vi "Auto Wheel Offsets.vi"() -> ()   [LabVIEW 2015]
uses:
  <vilib>/Rock Robotics/Network Tables/NT Write Number.vi
panel:
  out "FR Offset":dbl
  out "FL Offset":dbl
  out "BR Offset":dbl
  out "BL Offset":dbl
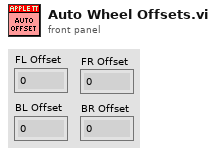
[diagram p1: front panel]
types:
  T1 = typedef "WPI_AnalogChannelDevRef.ctl" = cluster{"DevStatus":errorcluster, "Analog Channel":T2}
  T2 = typedef "FPGA_AIChannel.ctl" = enum8{"AI 0", "AI 1", "AI 2", "AI 3", "AI MXP 0", "AI MXP 1", "AI MXP 2", "AI MXP 3", "Invalid"}
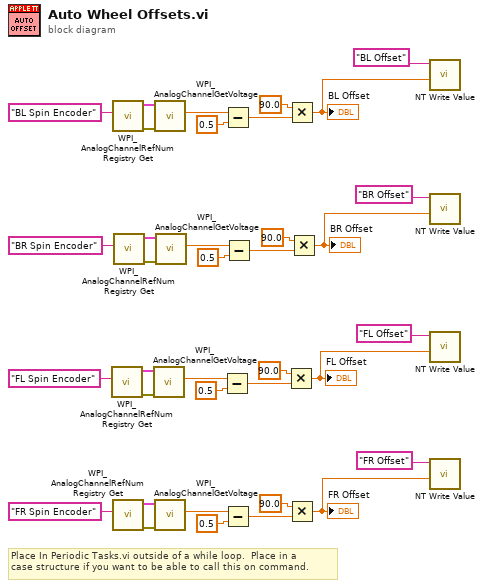
[diagram p0: block diagram]
diagram:
  # "Place In Periodic Tasks.vi outside of a while loop.  Place in a \ncase structure if you want to be able to call this on command."
  n1 = call <vilib>:"WPI_AnalogChannelRefNum Registry Get.vi"("refnum name"="FL Spin Encoder") -> ("error out"=w3:errorcluster, "AIDeviceRef"=w14:T1)  [unwired: 9 in]
  n2 = call <vilib>:"WPI_AnalogChannelRefNum Registry Get.vi"("refnum name"="BL Spin Encoder") -> ("error out"=w1:errorcluster, "AIDeviceRef"=w35:T1)  [unwired: 9 in]
  n3 = call <vilib>:"WPI_AnalogChannelRefNum Registry Get.vi"("refnum name"="FR Spin Encoder") -> ("error out"=w4:errorcluster, "AIDeviceRef"=w23:T1)  [unwired: 9 in]
  n4 = call <vilib>:"WPI_AnalogChannelRefNum Registry Get.vi"("refnum name"="BR Spin Encoder") -> ("error out"=w2:errorcluster, "AIDeviceRef"=w26:T1)  [unwired: 9 in]
  n5 = call <vilib>:"WPI_AnalogChannelGetVoltage.vi"("error in (no error)"=w3, "AIDeviceRef"=w14) -> ("Voltage"=w15:dbl)  [unwired: 7 in, 2 out]
  n6 = call <vilib>:"WPI_AnalogChannelGetVoltage.vi"("error in (no error)"=w1, "AIDeviceRef"=w35) -> ("Voltage"=w34:dbl)  [unwired: 7 in, 2 out]
  n7 = call <vilib>:"WPI_AnalogChannelGetVoltage.vi"("error in (no error)"=w4, "AIDeviceRef"=w23) -> ("Voltage"=w22:dbl)  [unwired: 7 in, 2 out]
  n8 = call <vilib>:"WPI_AnalogChannelGetVoltage.vi"("error in (no error)"=w2, "AIDeviceRef"=w26) -> ("Voltage"=w27:dbl)  [unwired: 7 in, 2 out]
  n9 = Subtract(x=w15, y=0.5) -> (x-y=w16:dbl)
  n10 = Subtract(x=w34, y=0.5) -> (x-y=w33:dbl)
  n11 = Subtract(x=w22, y=0.5) -> (x-y=w21:dbl)
  n12 = Subtract(x=w27, y=0.5) -> (x-y=w28:dbl)
  n13 = Multiply(x=90.0 ("y"), y=w16) -> (x*y=w8:dbl)
  "FL Offset" <- w8
  n14 = Multiply(x=90.0 ("y"), y=w33) -> (x*y=w6:dbl)
  "BL Offset" <- w6
  n15 = Multiply(x=90.0 ("y"), y=w21) -> (x*y=w7:dbl)
  "FR Offset" <- w7
  n16 = Multiply(x=90.0 ("y"), y=w28) -> (x*y=w5:dbl)
  "BR Offset" <- w5
  n17 = call-poly <vilib>:"NT Write Value.vi"("Numeric"=w6, "Name"="BL Offset") -> ()  [unwired: 9 in, 1 out]
  n18 = call-poly <vilib>:"NT Write Value.vi"("Numeric"=w5, "Name"="BR Offset") -> ()  [unwired: 9 in, 1 out]
  n19 = call-poly <vilib>:"NT Write Value.vi"("Numeric"=w8, "Name"="FL Offset") -> ()  [unwired: 9 in, 1 out]
  n20 = call-poly <vilib>:"NT Write Value.vi"("Numeric"=w7, "Name"="FR Offset") -> ()  [unwired: 9 in, 1 out]
